vi "SetPositionPIDigital.vi"(1 "Current Position (µm) 2":cluster{"x":dbl, "y":dbl, "z":dbl} caption="Current Position (µm)" {"z" format="%.2f"; "y" format="%.2f"; "x" format="%.2f"}) -> (0 "error out 2":errorcluster)   [LabVIEW 2009]
panel:
  out "Velocity":dbl[](array[numeric]) format="%.6f"
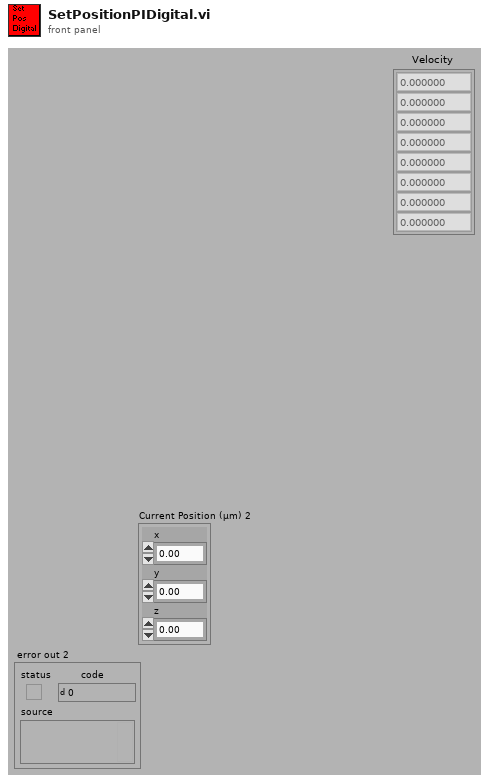
[diagram p1: front panel]
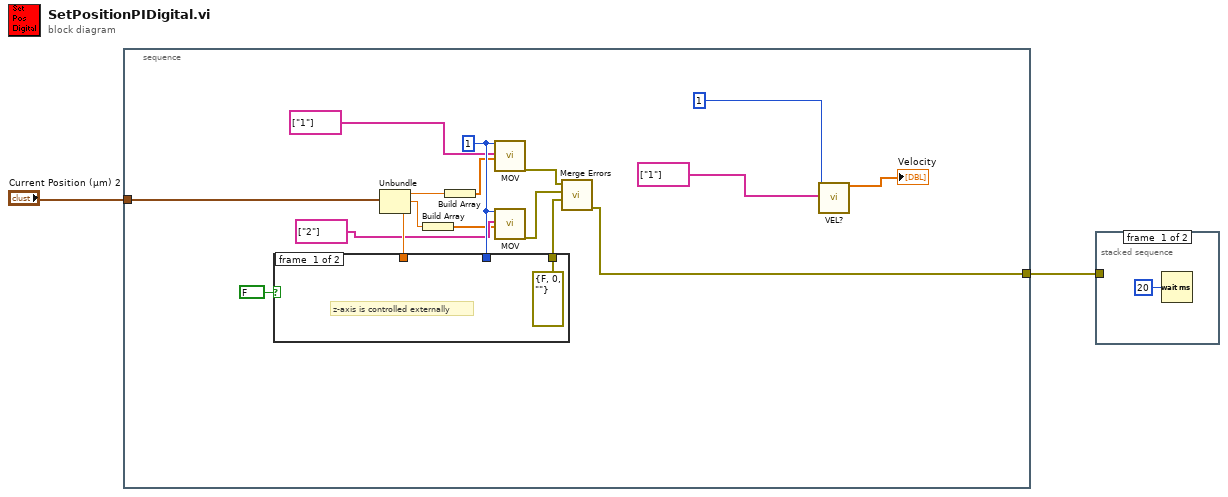
[diagram p0: block diagram]
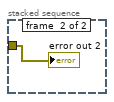
[diagram p2: hidden frame]
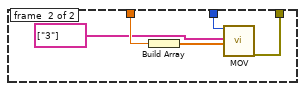
[diagram p3: hidden frame]
diagram:
  n1 = stacked-sequence {
    tunnel: "Current Position (µm) 2" -> [w9]
    tunnel: [w8] -> w1
    frame #0 {
      w16 = 1 ("System no.")
      n2 = Unbundle(w9) -> ("x"=w19:dbl, "y"=w18:dbl, "z"=w17:dbl)
      n3 = case shown="False" FALSE {
        tunnel: w17 -> [_ w25]
        tunnel: w16 -> [_ w23]
        tunnel: [errorcluster {"status"=FALSE, "code"=0, "source"=""} ("error out") w21] -> w11
        frame #0 {
          # "z-axis is controlled externally"
        }
        frame #1 {
          n4 = Build Array(w25) -> (w24:dbl[])
          n5 = call "MOV.vi"("System no."=w23, "Axes to move"=string[] ["3"], "Position values"=w24) -> ("error out"=w21:errorcluster)  [unwired: 16 in]
        }
      }
      n6 = Build Array(w18) -> (w6:dbl[])
      n7 = Build Array(w19) -> (w7:dbl[])
      n8 = call "MOV.vi"("System no."=w16, "Axes to move"=string[] ["1"], "Position values"=w7) -> ("error out"=w13:errorcluster)  [unwired: 16 in]
      n9 = call "MOV.vi"("System no."=w16, "Axes to move"=string[] ["2"], "Position values"=w6) -> ("error out"=w12:errorcluster)  [unwired: 16 in]
      n10 = call <vilib>:"Merge Errors.vi"("error in 3 (no error)"=w11, "error in 2 (no error)"=w12, "error in 1 (no error)"=w13) -> ("error out"=w8:errorcluster)  [unwired: 4 in]
      n11 = call "VEL?.vi"("System no."=1, "Axes to query"=string[] ["1"] ("Axes to move")) -> ("Velocity"=→"Velocity":dbl[])  [unwired: 16 in, 1 out]
    }
  }
  n12 = stacked-sequence {
    tunnel: w1 -> [_ w27]
    frame #0 {
      n13 = Wait (ms)(milliseconds to wait=u32 20) -> ()  [unwired: 1 out]
    }
    frame #1 {
      "error out 2" <- w27
    }
  }
